vi "Aenderung bei Rezeptwechsel.vi"(6 "Enum":T1, 8 "error in (no error)":errorcluster caption="Fehler (Eingang, kein Fehler)") -> (0 "error out":errorcluster caption="Fehler (Ausgang)")   [LabVIEW 2020, in "Erweiterte Konfig.lvlib" / "CG-Check Konfig.lvlib"]
uses:
  CG-Check Konfig.lvlib
  Aktion Aenderung bei Rezeptwechsel.ctl
  Aktion_CG-Check.ctl
  AK-Schnittstelle/AK Namen Aktionen.ctl
  AK-Schnittstelle/AK-Schnittstelle.lvlib
panel:
  out "MG Eingang":string[](array[string])
  out "Span3":string[](array[string])
  out "Span2":string[](array[string])
  out "Span1":string[](array[string])
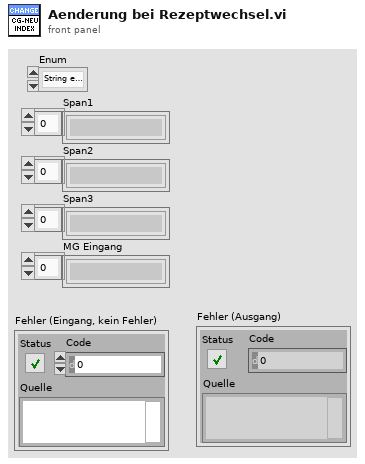
[diagram p1: front panel]
types:
  T1 = typedef "Erweiterte Konfig.lvlib/CG-Check Konfig.lvlib/Aktion Aenderung bei Rezeptwechsel.ctl" = enum16{"String erzeugen", "Index erzeugen"}
  T2 = typedef "AK-Schnittstelle.lvlib/AK Namen Aktionen.ctl" = enum16{"lesen", "laden", "speichern Namen", "AK Namen", "Liste erstellen", "EKFG erstellen", "speichern EKFG", "EKFG schreiben", "Neuen Eintrag erzeugen"}
  T3 = typedef "Erweiterte Konfig.lvlib/CG-Check Konfig.lvlib/Aktion_CG-Check.ctl" = enum16{"lesen", "schreiben", "laden", "Komponente", "Aktive?", "speichern"}
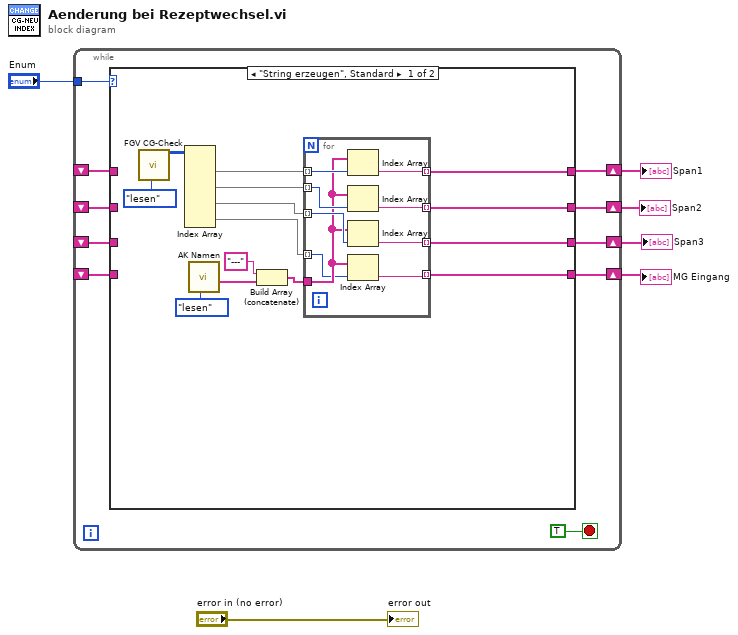
[diagram p0: block diagram]
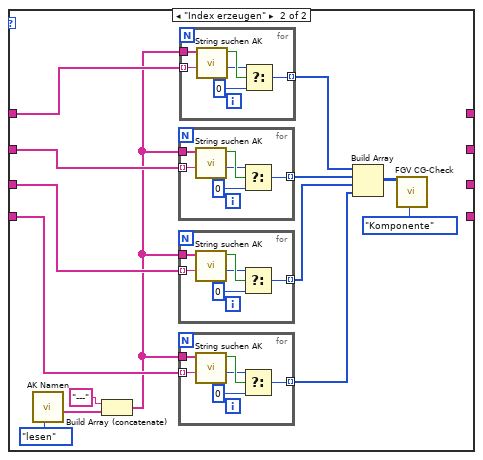
[diagram p2: hidden frame]
diagram:
  n1 = while {
    tunnel: "Enum" -> [w15]
    shift-right: [w14] -> w5
    shift-left: _ -> [w10]
    shift-right: [w13] -> w4
    shift-left: _ -> [w9]
    shift-right: [w12] -> w3
    shift-left: _ -> [w8]
    shift-right: [w11] -> w2
    shift-left: _ -> [w7]
    stop <- TRUE stop-if-true
    n2 = case shown="\"String erzeugen\", Standard" w15 {
      tunnel: [w22 _] -> w14
      tunnel: [w21 _] -> w13
      tunnel: [w20 _] -> w12
      tunnel: [w19 _] -> w11
      tunnel: w10 -> [_ w49]
      tunnel: w9 -> [_ w48]
      tunnel: w8 -> [_ w47]
      tunnel: w7 -> [_ w46]
      frame "String erzeugen", Default {
        n3 = call "FGV CG-Check.vi"("Aktion"=Aktion_CG-Check."lesen") -> ("Komponenten"=w29:u16[][])  [unwired: 11 in, 7 out]
        n4 = Index Array(array=w29) -> (element #1=w25:u16[], element #2=w28:u16[], element #3=w27:u16[], element #4=w23:u16[])  [unwired: 8 in]
        n5 = call "AK Namen.vi"("Aktionen"=AK_Namen_Aktionen."lesen") -> ("AK Namen"=w24:string[])  [unwired: 7 in, 3 out]
        n6 = Build Array (concatenate)("---" ("String"), w24) -> (w18:string[])
        n7 = for {
          tunnel: w25 -> [w39] mode=indexing
          tunnel: w28 -> [w38] mode=indexing
          tunnel: w27 -> [w37] mode=indexing
          tunnel: w18 -> [w32]
          tunnel: [w36] -> w22 mode=indexing
          tunnel: [w35] -> w21 mode=indexing
          tunnel: [w34] -> w20 mode=indexing
          tunnel: [w33] -> w19 mode=indexing
          tunnel: w23 -> [w31] mode=indexing
          n8 = Index Array(array=w32, index=w39) -> (element=w36:string)
          n9 = Index Array(array=w32, index=w38) -> (element=w35:string)
          n10 = Index Array(array=w32, index=w37) -> (element=w34:string)
          n11 = Index Array(array=w32, index=w31) -> (element=w33:string)
        }
      }
      frame "Index erzeugen" {
        n12 = call "AK Namen.vi"("Aktionen"=AK_Namen_Aktionen."lesen") -> ("AK Namen"=w52:string[])  [unwired: 7 in, 3 out]
        n13 = Build Array (concatenate)("---" ("String"), w52) -> (w41:string[])
        n14 = for {
          tunnel: w48 -> [w70] mode=indexing
          tunnel: [w67] -> w44 mode=indexing
          tunnel: w41 -> [w71]
          n15 = call "String suchen AK.vi"("gesucht"=w70, "Namen"=w71) -> ("Index"=w68:i32, "Gefunden?"=w69:bool)  [unwired: 8 in]
          n16 = Select(t=w68, s=w69, f=0) -> (s? t:f=w67:i32)
        }
        n17 = for {
          tunnel: w47 -> [w64] mode=indexing
          tunnel: [w61] -> w43 mode=indexing
          tunnel: w41 -> [w65]
          n18 = call "String suchen AK.vi"("gesucht"=w64, "Namen"=w65) -> ("Index"=w62:i32, "Gefunden?"=w63:bool)  [unwired: 8 in]
          n19 = Select(t=w62, s=w63, f=0) -> (s? t:f=w61:i32)
        }
        n20 = for {
          tunnel: w46 -> [w54] mode=indexing
          tunnel: [w56] -> w42 mode=indexing
          tunnel: w41 -> [w59]
          n21 = call "String suchen AK.vi"("gesucht"=w54, "Namen"=w59) -> ("Index"=w57:i32, "Gefunden?"=w58:bool)  [unwired: 8 in]
          n22 = Select(t=w57, s=w58, f=0) -> (s? t:f=w56:i32)
        }
        n23 = for {
          tunnel: w49 -> [w76] mode=indexing
          tunnel: [w73] -> w45 mode=indexing
          tunnel: w41 -> [w77]
          n24 = call "String suchen AK.vi"("gesucht"=w76, "Namen"=w77) -> ("Index"=w74:i32, "Gefunden?"=w75:bool)  [unwired: 8 in]
          n25 = Select(t=w74, s=w75, f=0) -> (s? t:f=w73:i32)
        }
        n26 = Build Array(w45, w44, w43, w42) -> (w50:i32[][])
        n27 = call "FGV CG-Check.vi"("Komponenten"=w50, "Aktion"=Aktion_CG-Check."Komponente") -> ()  [unwired: 10 in, 8 out]
      }
    }
  }
  "Span1" <- w5
  "Span2" <- w4
  "Span3" <- w3
  "MG Eingang" <- w2
  "error out" <- "error in (no error)"
